vi "Create Goals.vi"(8 "error in (no error)":errorcluster, 9 "Current Month":T1, 10 "Current YYYY":i32, 11 "Database in":refnum<class "Account History.lvclass">) -> (0 "error out":errorcluster, 3 "Database out":refnum<class "Account History.lvclass">)   [LabVIEW 2018, in "Account History.lvclass"]
uses:
  Account History.lvclass
  Month.ctl
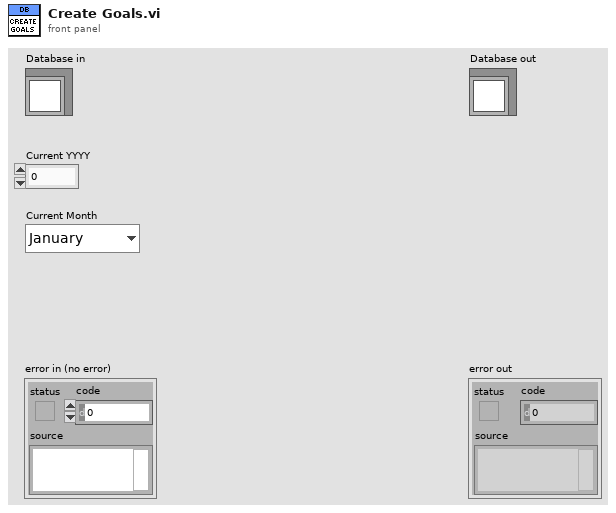
[diagram p1: front panel]
types:
  T1 = typedef "Account History.lvclass/Month.ctl" = enum16{"January", "February", "March", "April", "May", "June", "July", "August", "September", "October", "November", "December"}
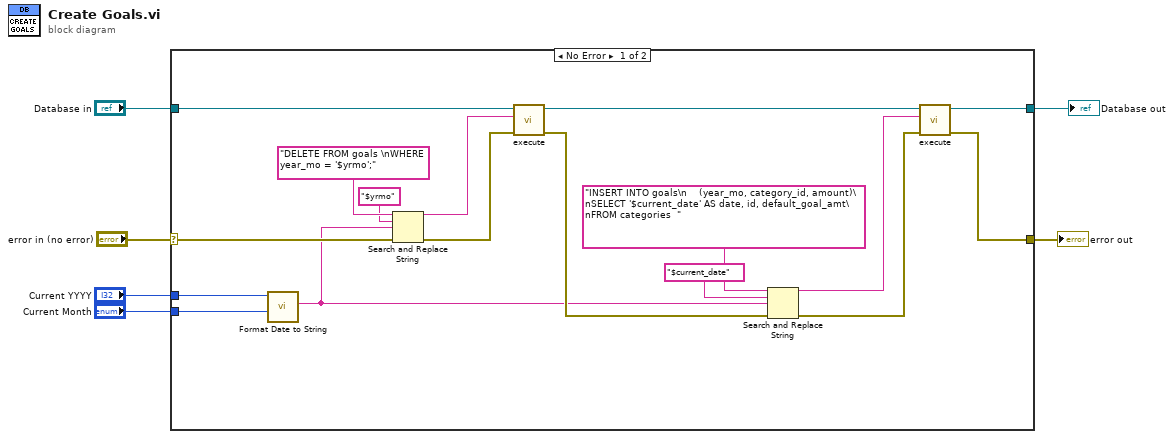
[diagram p0: block diagram]
diagram:
  n1 = case shown="No Error" "error in (no error)" {
    selector: "error in (no error)" -> [w21 w25]
    tunnel: [w20 w25] -> w5
    tunnel: [w22 w24] -> w3
    tunnel: "Database in" -> [w23 w24]
    tunnel: "Current YYYY" -> [w19 _]
    tunnel: "Current Month" -> [w18 _]
    frame No Error {
      n2 = call "Format Date to String.vi"("Month"=w18, "YYYY"=w19) -> ("Year-Mo"=w10:string)  [unwired: 9 in]
      n3 = Search and Replace String(input string="DELETE FROM goals \nWHERE year_mo = '$yrmo';", search string="$yrmo", replace string=w10, error in=w21) -> (result string=w15:string, error out=w14:errorcluster)  [unwired: 4 in, 2 out]
      n4 = call "execute.vi"("error in (no error)"=w14, "SQL query"=w15, "Database in"=w23) -> ("error out"=w11:errorcluster, "Database out"=w13:refnum<class "Account History.lvclass">)  [unwired: 7 in]
      n5 = Search and Replace String(input string="INSERT INTO goals\n    (year_mo, category_id, amount)\nSELECT '$current_date' AS date, id, default_goal_amt\nFROM categories  ", search string="$current_date", replace string=w10, error in=w11) -> (result string=w9:string, error out=w8:errorcluster)  [unwired: 4 in, 2 out]
      n6 = call "execute.vi"("error in (no error)"=w8, "SQL query"=w9, "Database in"=w13) -> ("error out"=w20:errorcluster, "Database out"=w22:refnum<class "Account History.lvclass">)  [unwired: 7 in]
    }
    frame Error {
    }
  }
  "error out" <- w5
  "Database out" <- w3
